vi "data to acc_gyro_sync.vi"(0 "byte array":u8[](array[numeric]), 1 "gyro range (deg/s)":dbl=250.0, 2 "accel range (m/s2)":dbl=8.0) -> (3 "acc gyro data":T1)   [LabVIEW 2013]
uses:
  acc_gyro_sync_data.ctl
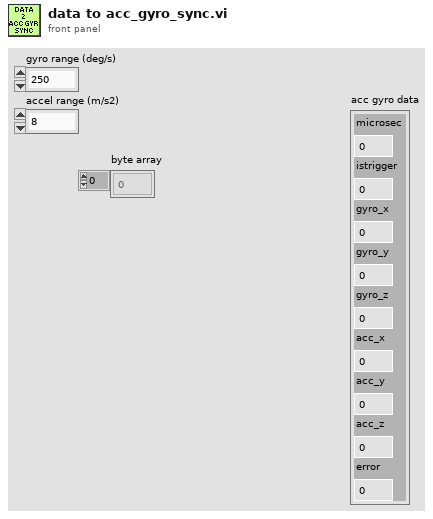
[diagram p1: front panel]
types:
  T1 = typedef "acc_gyro_sync_data.ctl" = cluster{"microsec":u32, "istrigger":u8, "gyro_x":dbl, "gyro_y":dbl, "gyro_z":dbl, "acc_x":dbl, "acc_y":dbl, "acc_z":dbl, "error":u32}
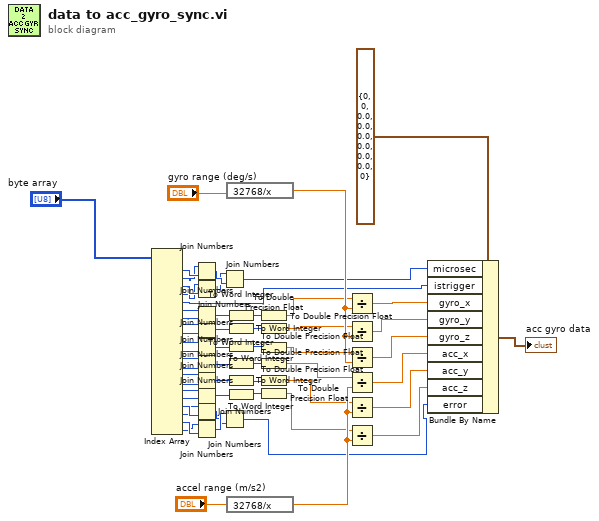
[diagram p0: block diagram]
diagram:
  n1 = Index Array(array="byte array") -> (element #1=w13:u8, element #2=w12:u8, element #3=w11:u8, element #4=w10:u8, element #5=w9:u8, element #6=w57:u8, element #7=w56:u8, element #8=w55:u8, element #9=w54:u8, element #10=w53:u8, element #11=w52:u8, element #12=w51:u8, element #13=w50:u8, element #14=w49:u8, element #15=w48:u8, element #16=w47:u8, element #17=w46:u8, element #18=w5:u8, element #19=w4:u8, element #20=w3:u8, element #21=w2:u8)  [unwired: 21 in]
  n2 = Join Numbers(hi=w12, lo=w13) -> ((hi.lo)=w16:u16)
  n3 = Join Numbers(hi=w10, lo=w11) -> ((hi.lo)=w15:u16)
  n4 = Join Numbers(hi=w57, lo=w56) -> ((hi.lo)=w45:u16)
  n5 = Join Numbers(hi=w55, lo=w54) -> ((hi.lo)=w44:u16)
  n6 = Join Numbers(hi=w53, lo=w52) -> ((hi.lo)=w43:u16)
  n7 = Join Numbers(hi=w51, lo=w50) -> ((hi.lo)=w42:u16)
  n8 = Join Numbers(hi=w49, lo=w48) -> ((hi.lo)=w41:u16)
  n9 = Join Numbers(hi=w47, lo=w46) -> ((hi.lo)=w40:u16)
  n10 = Join Numbers(hi=w4, lo=w5) -> ((hi.lo)=w6:u16)
  n11 = Join Numbers(hi=w2, lo=w3) -> ((hi.lo)=w7:u16)
  n12 = Join Numbers(hi=w15, lo=w16) -> ((hi.lo)=w8:u32)
  n13 = Join Numbers(hi=w7, lo=w6) -> ((hi.lo)=w1:u32)
  n14 = To Word Integer(number=w45) -> (16bit integer=w39:i16)
  n15 = To Word Integer(number=w44) -> (16bit integer=w38:i16)
  n16 = To Word Integer(number=w43) -> (16bit integer=w37:i16)
  n17 = To Word Integer(number=w42) -> (16bit integer=w36:i16)
  n18 = To Word Integer(number=w41) -> (16bit integer=w35:i16)
  n19 = To Word Integer(number=w40) -> (16bit integer=w34:i16)
  n20 = expression code="32768/x"("gyro range (deg/s)") -> (w23:dbl)
  n21 = expression code="32768/x"("accel range (m/s2)") -> (w25:dbl)
  n22 = To Double Precision Float(number=w39) -> (double precision float=w22:dbl)
  n23 = To Double Precision Float(number=w38) -> (double precision float=w21:dbl)
  n24 = To Double Precision Float(number=w37) -> (double precision float=w20:dbl)
  n25 = To Double Precision Float(number=w36) -> (double precision float=w19:dbl)
  n26 = To Double Precision Float(number=w35) -> (double precision float=w18:dbl)
  n27 = To Double Precision Float(number=w34) -> (double precision float=w17:dbl)
  n28 = Divide(x=w22, y=w23) -> (x/y=w14:dbl)
  n29 = Divide(x=w21, y=w23) -> (x/y=w33:dbl)
  n30 = Divide(x=w20, y=w23) -> (x/y=w32:dbl)
  n31 = Divide(x=w19, y=w25) -> (x/y=w31:dbl)
  n32 = Divide(x=w18, y=w25) -> (x/y=w30:dbl)
  n33 = Divide(x=w17, y=w25) -> (x/y=w29:dbl)
  n34 = Bundle By Name(cluster=T1 {"microsec"=0, "istrigger"=0, "gyro_x"=0.0, "gyro_y"=0.0, "gyro_z"=0.0, "acc_x"=0.0, "acc_y"=0.0, "acc_z"=0.0, "error"=0} ("acc gyro data 2"), "microsec"=w8, "istrigger"=w9, "gyro_x"=w14, "gyro_y"=w33, "gyro_z"=w32, "acc_x"=w31, "acc_y"=w30, "acc_z"=w29, "error"=w1) -> (→"acc gyro data":T1)
